vi "Reference FPGA X410.vi"() -> ()   [LabVIEW 2025]
doc: "this VI is the top level of the FPGA.\n\nsubVIs placed at this level:\nmust have fixed-sized arrays.\ncontaining a class input (control) must NOT be left unconnected.\n\nconditional symbols supported for ease-of-use in building variations of the image are documented in a comment section and should be kept up-to-date."
uses:
  <vilib>/Platform/TimedLoop/XDataNode/timing_clust.ctl
  <vilib>/Platform/TimedLoop/XDataNode/nitl_modes.ctl
  <vilib>/Platform/TimedLoop/XDataNode/wakeup.ctl
  <vilib>/rvi/Emulation/niFpgaSctlEmulationGetInTimedLoop.vi
  <vilib>/rvi/Emulation/niFpgaEmulationReportErrorSimple.vi
  <vilib>/rvi/Emulation/niFpgaGetClockAttributes.vi
  <vilib>/rvi/Emulation/niFpgaCriticalErrorInLSC.vi
  <vilib>/Platform/TimedLoop/XDataNode/XDataNode.xnode
  Instruction Framework/niUSRP Reference FPGA v1.lvclass
  Rx DSP/niUSRP Rx DSP v2 FPGA.lvclass
  Rx Core/niUSRP Rx Core v1 FPGA.lvclass
  Sync/niUSRP Rx Core v1 FPGA/niUSRP Sync v1 FPGA.lvclass
  Tx DSP/niUSRP Tx DSP v2 FPGA.lvclass
  <vilib>/Platform/TimedLoop/XDataNode/XDNodeRunTimeDep.lvlib
  Stream Control/niUSRP Stream Control (DMA) v1 FPGA.lvclass
  <instrlib>/_niInstr/FIFO Register Bus/v1/FPGA/niInstr FIFO Register Bus v1 FPGA.lvclass
  <instrlib>/_niInstr/Instruction Framework/v1/FPGA/Collection Builder/Collection Builder.lvclass
  Tx Core/niUSRP Tx Core v1 FPGA.lvclass
panel:
  out "fifo reg bus data 0":u64
  out "fifo reg bus status 0":u32
  in  "fifo reg bus ctrl 0":u32
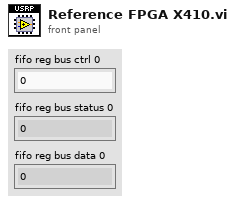
[diagram p1: front panel]
types:
  T1 = typedef "XDNodeRunTimeDep.lvlib/timing_clust.ctl" = cluster{"Expected End [f-1]":u64, "Actual End [f-1]":u64, "Finished Late? [f-1]":bool, "Expected End [i-1]":u64, "Actual End [i-1]":u64, "Finished Late? [i-1]":bool, "Expected Start [i]":u64, "Actual Start [i]":u64, "Expected Start [f]":u64, "Actual Start [f]":u64, "Source Name":string, "Structure Name":string, "Period":i64, "Deadline":i64, "Offset":i64, "Start":i64, "Priority":i32, "Timeout":i32, "Mode":T2, "Wakeup Reason":T3, "Error":errorcluster, "Source Type":string, "Secondary Source Type":string, "Global End Time":u64, "Global Start Time":u64, "Frame Duration":u64, "Iteration Duration":u64, "Assigned CPU":i32, "I/O Scan Engine Mode":u32}
  T2 = typedef "XDNodeRunTimeDep.lvlib/nitl_modes.ctl" = enum32{"No Change", "Process missed periods, maintain original phase", "Discard missed periods, maintain original phase", "Process missed periods, ignore original phase", "Discard missed periods, ignore original phase"}
  T3 = typedef "XDNodeRunTimeDep.lvlib/wakeup.ctl" = enum32{"Normal", "Aborted", "Asynchronous wakeup", "Timing source error", "Timed loop error", "Timeout"}
  T4 = typedef "niInstr DSP v1 Shared.lvlib/IQ Data.ctl" = cluster{"I":fxp<+/-,18,1>, "Q":fxp<+/-,18,1>, "overflow":bool}
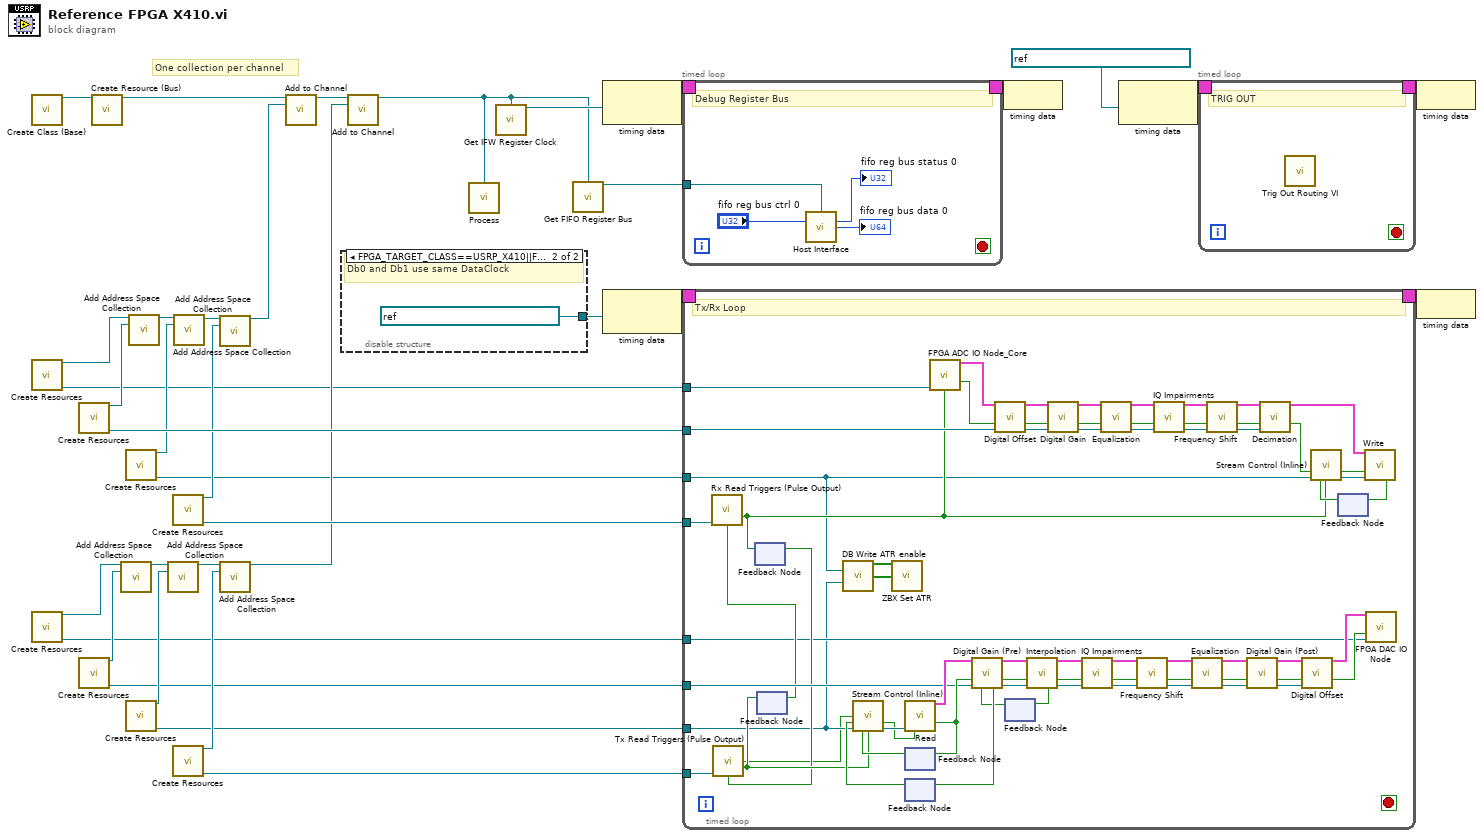
[diagram p0: block diagram]
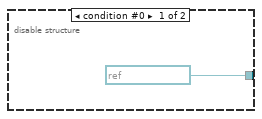
[diagram p2: hidden frame]
diagram:
  # "One collection per channel"
  n1 = call "Create Class (Base).vi"() -> ("reference fpga"=w34:refnum<class "niUSRP Reference FPGA v1.lvclass">)  [unwired: 15 in]
  n2 = call "Create Resources.vi"() -> ("channel collection builder"=w26:refnum<class "Collection Builder.lvclass">, "niVST Common Reference FPGA.lvclass"=w5:refnum<class "niUSRP Rx Core v1 FPGA.lvclass">)  [unwired: 14 in]
  n3 = call "Create Resources.vi"() -> ("channel collection builder"=w18:refnum<class "Collection Builder.lvclass">, "niUSRP Tx Core"=w8:refnum<class "niUSRP Tx Core v1 FPGA.lvclass">)  [unwired: 14 in]
  n4 = call "Create Resources.vi"() -> ("address space collection"=w30:refnum<class "Address Space Collection.lvclass">, "acq dsp session"=w31:refnum<class "niUSRP Rx DSP v2 FPGA.lvclass">)  [unwired: 14 in]
  n5 = call "Create Resources.vi"() -> ("address space collection"=w17:refnum<class "Address Space Collection.lvclass">, "tx dsp"=w10:refnum<class "niUSRP Tx DSP v2 FPGA.lvclass">)  [unwired: 14 in]
  n6 = call-dynamic "Create Resource (Bus).vi"("reference fpga in"=w34) -> ("reference fpga out"=w29:refnum<class "niUSRP Reference FPGA v1.lvclass">)  [unwired: 14 in]
  n7 = call <instrlib>:"Add Address Space Collection.vi"("collection builder in"=w18, "address space collection"=w17) -> ("collection builder out"=w16:refnum<class "Collection Builder.lvclass">)  [unwired: 13 in]
  n8 = call "Create Resources.vi"() -> ("address space collection"=w13:refnum<class "Address Space Collection.lvclass">, "stream session"=w7:refnum<class "niUSRP Stream Control (DMA) v1 FPGA.lvclass">)  [unwired: 14 in]
  n9 = call "Create Resources.vi"() -> ("address space collection"=w20:refnum<class "Address Space Collection.lvclass">, "stream session"=w6:refnum<class "niUSRP Stream Control (DMA) v1 FPGA.lvclass">)  [unwired: 14 in]
  n10 = call <instrlib>:"Add Address Space Collection.vi"("collection builder in"=w26, "address space collection"=w30) -> ("collection builder out"=w28:refnum<class "Collection Builder.lvclass">)  [unwired: 13 in]
  n11 = call <instrlib>:"Add Address Space Collection.vi"("collection builder in"=w16, "address space collection"=w20) -> ("collection builder out"=w22:refnum<class "Collection Builder.lvclass">)  [unwired: 13 in]
  n12 = call "Create Resources.vi"() -> ("address space collection"=w12:refnum<class "Address Space Collection.lvclass">, "stream control session"=w27:refnum<class "niUSRP Sync v1 FPGA.lvclass">)  [unwired: 14 in]
  n13 = call "Create Resources.vi"() -> ("address space collection"=w19:refnum<class "Address Space Collection.lvclass">, "stream control session"=w9:refnum<class "niUSRP Sync v1 FPGA.lvclass">)  [unwired: 14 in]
  n14 = call <instrlib>:"Add Address Space Collection.vi"("collection builder in"=w28, "address space collection"=w13) -> ("collection builder out"=w25:refnum<class "Collection Builder.lvclass">)  [unwired: 13 in]
  n15 = call <instrlib>:"Add Address Space Collection.vi"("collection builder in"=w25, "address space collection"=w12) -> ("collection builder out"=w24:refnum<class "Collection Builder.lvclass">)  [unwired: 13 in]
  n16 = call <instrlib>:"Add Address Space Collection.vi"("collection builder in"=w22, "address space collection"=w19) -> ("collection builder out"=w21:refnum<class "Collection Builder.lvclass">)  [unwired: 13 in]
  n17 = call-dynamic "Add to Channel.vi"("reference fpga in"=w29, "collection builder in"=w24) -> ("reference fpga out"=w23:refnum<class "niUSRP Reference FPGA v1.lvclass">)  [unwired: 13 in]
  n18 = disable-structure shown="FPGA_TARGET_CLASS==USRP_X410||FPGA_TARGET_CLASS==USRP_X410__EMBEDDED____UNSUPPORTED" {
    disable-tunnel: [refnum<k21> "Data Clock" ("Source Name") refnum<k21> "Daughterboard 0\\Data Clock" ("Source Name")] -> w2
    frame condition #0 {
    }
    frame condition #1 (active) {
      # "Db0 and Db1 use same DataClock"
    }
  }
  n19 = call-dynamic "Add to Channel.vi"("reference fpga in"=w23, "collection builder in"=w21) -> ("reference fpga out"=w11:refnum<class "niUSRP Reference FPGA v1.lvclass">)  [unwired: 13 in]
  n20 = call "Process.vi"("reference fpga"=w11) -> ()  [unwired: 15 in]
  n21 = call-dynamic "Get IFW Register Clock.vi"("reference fpga"=w11) -> ("ifw register clock"=w32:refnum<k21>)  [unwired: 14 in]
  n22 = call-dynamic "Get FIFO Register Bus.vi"("reference fpga"=w11) -> ("fifo register bus"=w33:refnum<class "niInstr FIFO Register Bus v1 FPGA.lvclass">)  [unwired: 14 in]
  n23 = node-c288 ("Input Node")(w32) -> (w36:T1)
  n24 = node-c288(w2) -> (w15:T1)
  n25 = timed-loop {
    timing: w36 -> [_]
    timing-out: [_] -> w35
    tunnel: w33 -> [w39]
    stop <- _ stop-if-true
    # "Debug Register Bus"
    n26 = call <instrlib>:"Host Interface.vi"("fifo register bus"=w39, "fifo reg bus ctrl 0"="fifo reg bus ctrl 0") -> ("fifo reg bus status 0"=→"fifo reg bus status 0":u32, "fifo reg bus data 0"=→"fifo reg bus data 0":u64)  [unwired: 12 in]
  }
  n27 = timed-loop "Acquisition Loop" {
    timing: w15 -> [_]
    timing-out: [_] -> w14
    tunnel: w31 -> [w102]
    tunnel: w5 -> [w51]
    tunnel: w27 -> [w98]
    tunnel: w7 -> [w47]
    tunnel: w8 -> [w50]
    tunnel: w10 -> [w63]
    tunnel: w6 -> [w46]
    tunnel: w9 -> [w62]
    stop <- _ stop-if-true
    # "Tx/Rx Loop"
    n28 = feedback #1() -> (w58:bool)  [unwired: 1 in]
    n29 = call-dynamic "Tx Read Triggers (Pulse Output).vi"("niUSRP Sync"=w62, "external trigger"=w58) -> ("future trigger"=w45:bool, "output valid"=w61:bool)  [unwired: 10 in, 2 out]
    n30 = feedback #2() -> (w59:bool)  [unwired: 1 in]
    n31 = call-dynamic "Rx Read Triggers (Pulse Output).vi"("niUSRP Sync"=w98, "external trigger"=w59) -> ("output valid"=w60:bool)  [unwired: 11 in, 2 out]
    n32 = feedback-in #1(w60) -> ()
    n33 = feedback-in #2(w61) -> ()
    n34 = call "DB Write ATR enable.vi"("stream session rx"=w47, "stream session tx"=w46) -> ("db 0"=w49:bool[], "db1"=w48:bool[])  [unwired: 12 in]
    n35 = call "ZBX Set ATR.vi"("DB 1"=w48, "DB 0"=w49) -> ()  [unwired: 10 in]
    n36 = feedback #3() -> (w64:bool)  [unwired: 1 in]
    n37 = feedback #4() -> (w65:bool)  [unwired: 1 in]
    n38 = call "Stream Control (Inline).vi"("future trigger"=w45, "input valid"=w65, "stream control"=w46, "ready for output"=w64, "trigger"=w61) -> ("stream"=w67:bool, "stream control"=w74:refnum<class "niUSRP Stream Control (DMA) v1 FPGA.lvclass">)  [unwired: 7 in, 2 out]
    n39 = call "Read.vi"("stream control"=w74, "ready for output"=w67) -> ("data out"=w76:T4[], "output valid"=w66:bool)  [unwired: 11 in, 1 out]
    n40 = feedback-in #3(w66) -> ()
    n41 = call-dynamic "FPGA ADC IO Node_Core.vi"("rx core"=w51, "trigger"=w60) -> ("data"=w88:T4[], "output valid"=w87:bool)  [unwired: 10 in, 2 out]
    n42 = call-dynamic "Digital Offset.vi"("data in"=w88, "input valid"=w87, "acq in"=w102) -> ("data out"=w111:T4[], "output valid"=w110:bool, "acq out"=w109:refnum<class "niUSRP Rx DSP v2 FPGA.lvclass">)  [unwired: 9 in, 1 out]
    n43 = feedback #5() -> (w53:bool)  [unwired: 1 in]
    n44 = call-dynamic "Digital Gain (Pre).vi"("data in"=w76, "input valid"=w66, "gen in"=w63, "ready for output (T)"=w53) -> ("data out"=w55:T4[], "output valid"=w57:bool, "ready for input"=w75:bool, "gen out"=w56:refnum<class "niUSRP Tx DSP v2 FPGA.lvclass">)  [unwired: 8 in]
    n45 = feedback-in #4(w75) -> ()
    n46 = call-dynamic "Interpolation.vi"("data in"=w55, "input valid"=w57, "gen in"=w56) -> ("data out"=w85:T4[], "output valid"=w78:bool, "ready for input"=w54:bool, "gen out"=w77:refnum<class "niUSRP Tx DSP v2 FPGA.lvclass">)  [unwired: 9 in]
    n47 = feedback-in #5(w54) -> ()
    n48 = call-dynamic "Digital Gain.vi"("data in"=w111, "input valid"=w110, "acq in"=w109) -> ("data out"=w106:T4[], "output valid"=w107:bool, "acq out"=w108:refnum<class "niUSRP Rx DSP v2 FPGA.lvclass">)  [unwired: 9 in, 1 out]
    n49 = call-dynamic "IQ Impairments.vi"("data in"=w85, "input valid"=w78, "gen in"=w77) -> ("data out"=w73:T4[], "output valid"=w70:bool, "gen out"=w71:refnum<class "niUSRP Tx DSP v2 FPGA.lvclass">)  [unwired: 9 in, 1 out]
    n50 = call-dynamic "Equalization.vi"("data in"=w106, "input valid"=w107, "acq in"=w108) -> ("data out"=w105:T4[], "output valid"=w104:bool, "acq out"=w103:refnum<class "niUSRP Rx DSP v2 FPGA.lvclass">)  [unwired: 9 in, 1 out]
    n51 = call-dynamic "Frequency Shift.vi"("data in"=w73, "input valid"=w70, "gen in"=w71) -> ("data out"=w72:T4[], "output valid"=w69:bool, "gen out"=w68:refnum<class "niUSRP Tx DSP v2 FPGA.lvclass">)  [unwired: 9 in, 1 out]
    n52 = call-dynamic "IQ Impairments.vi"("data in"=w105, "input valid"=w104, "acq in"=w103) -> ("data out"=w97:T4[], "output valid"=w95:bool, "acq out"=w94:refnum<class "niUSRP Rx DSP v2 FPGA.lvclass">)  [unwired: 9 in, 1 out]
    n53 = call-dynamic "Equalization.vi"("data in"=w72, "input valid"=w69, "gen in"=w68) -> ("data out"=w84:T4[], "output valid"=w79:bool, "gen out"=w80:refnum<class "niUSRP Tx DSP v2 FPGA.lvclass">)  [unwired: 9 in, 1 out]
    n54 = call-dynamic "Frequency Shift.vi"("data in"=w97, "input valid"=w95, "acq in"=w94) -> ("data out"=w96:T4[], "output valid"=w92:bool, "acq out"=w93:refnum<class "niUSRP Rx DSP v2 FPGA.lvclass">)  [unwired: 9 in, 1 out]
    n55 = call-dynamic "Digital Gain (Post).vi"("data in"=w84, "input valid"=w79, "gen in"=w80) -> ("data out"=w83:T4[], "output valid"=w81:bool, "gen out"=w82:refnum<class "niUSRP Tx DSP v2 FPGA.lvclass">)  [unwired: 9 in, 1 out]
    n56 = call-dynamic "Decimation.vi"("data in"=w96, "input valid"=w92, "acq in"=w93) -> ("data out"=w89:T4[], "output valid"=w99:bool)  [unwired: 9 in, 2 out]
    n57 = call-dynamic "Digital Offset.vi"("data in"=w83, "input valid"=w81, "gen in"=w82) -> ("data out"=w52:T4[], "output valid"=w86:bool)  [unwired: 9 in, 2 out]
    n58 = feedback #6() -> (w90:bool)  [unwired: 1 in]
    n59 = call "Stream Control (Inline).vi"("input valid"=w99, "stream control"=w47, "ready for output"=w90, "trigger"=w60) -> ("stream"=w91:bool, "stream control"=w100:refnum<class "niUSRP Stream Control (DMA) v1 FPGA.lvclass">)  [unwired: 8 in, 2 out]
    n60 = call "Write.vi"("data in"=w89, "input valid"=w91, "stream control"=w100) -> ("ready for input"=w101:bool)  [unwired: 11 in, 1 out]
    n61 = feedback-in #6(w101) -> ()
    n62 = call "FPGA DAC IO Node.vi"("data"=w52, "input valid"=w86, "niUSRP Tx Core v1 FPGA.lvclass"=w50) -> ()  [unwired: 13 in]
  }
  n63 = node-c288(w35) -> ()
  n64 = node-c288 ("Input Node")(refnum<k21> "Daughterboard 0\\Data Clock" ("Source Name")) -> (w4:T1)
  n65 = timed-loop {
    timing: w4 -> [_]
    timing-out: [_] -> w3
    stop <- _ stop-if-true
    # "TRIG OUT"
    n66 = call "Trig Out Routing VI.vi"() -> ()  [unwired: 16 in]
  }
  n67 = node-c288(w3) -> ()
  n68 = node-c288(w14) -> ()
